vi "uSubscription IsAlive.vi"(8 "error in (no error)":errorcluster, 11 "uSubscription in":refnum<class "uSubscription.lvclass">) -> (0 "error out":errorcluster, 2 "Is Alive?":bool, 3 "uSubscription out":refnum<class "uSubscription.lvclass">)   [LabVIEW 2021, in "uFramework.lvlib" / "uSubscription.lvclass"]
uses:
  uSubscription.lvclass
  uSubscription.lvclass/uSubscription.ctl
  uTransport/uTransport.lvclass
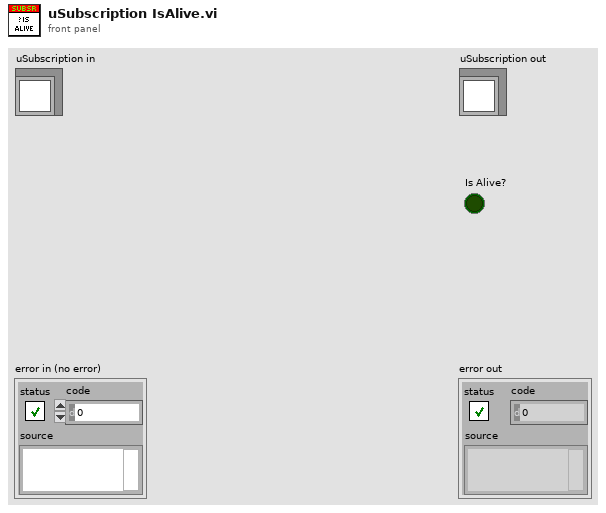
[diagram p1: front panel]
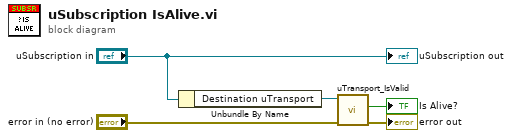
[diagram p0: block diagram]
diagram:
  n1 = Unbundle By Name("uSubscription in") -> ("Destination uTransport"=w4:refnum<class "uTransport.lvclass">)
  n2 = call-dynamic "uTransport_IsValid.vi"("error in (no error)"="error in (no error)", "uTransport in"=w4) -> ("error out"=→"error out":errorcluster, "IsValid?"=→"Is Alive?":bool)  [unwired: 7 in, 1 out]
  "uSubscription out" <- "uSubscription in"
